vi "Find Intersections of Hyperbolas.vi"(5 "Array":T1(array[cluster]), 9 "Domain":cluster{"Start":dbl, "Stop":dbl, "Step":dbl}={"Start"=-10.0, "Stop"=10.0, "Step"=0.1}) -> ()   [LabVIEW 2013]
uses:
  <vilib>/Analysis/baseanly.llb/A x Vector.vi
  <vilib>/gmath/NI_Gmath.lvlib
  <vilib>/Analysis/NI_AALBase.lvlib
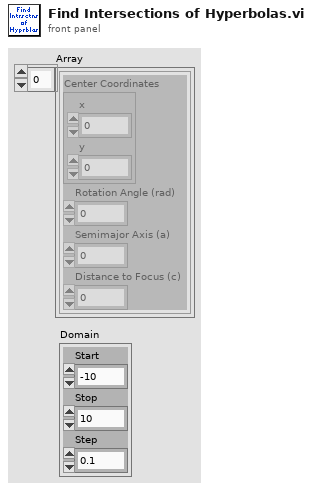
[diagram p1: front panel]
types:
  T1 = cluster{"Center Coordinates":cluster{"x":dbl, "y":dbl}, "Rotation Angle (rad)":dbl, "Semimajor Axis (a)":dbl, "Distance to Focus (c)":dbl}[]
  T2 = cluster{"A x Vector[0]":dbl, "A x Vector[1]":dbl}
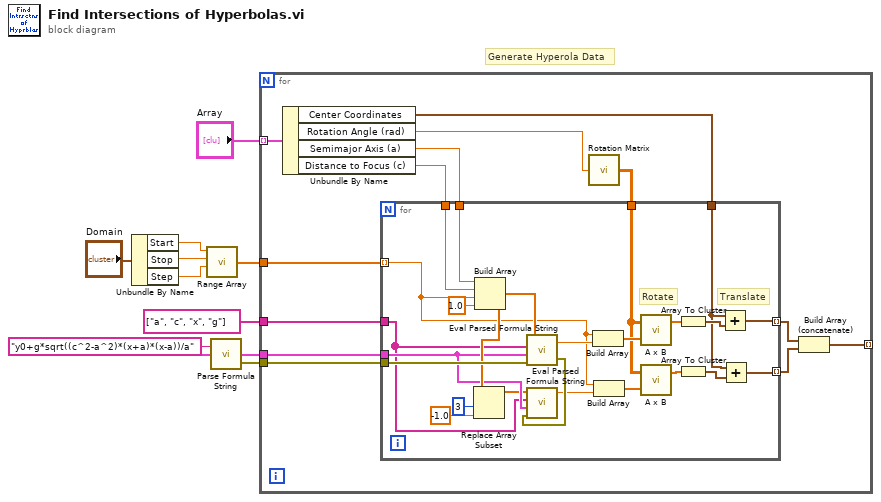
[diagram p0: block diagram]
diagram:
  # "Generate Hyperola Data"
  n1 = Unbundle By Name("Domain") -> ("Start"=w4:dbl, "Stop"=w3:dbl, "Step"=w2:dbl)
  n2 = call "Range Array.vi"("Step"=w2, "Stop"=w3, "Start"=w4) -> ("Range"=w7:dbl[])  [unwired: 3 in]
  n3 = call <vilib>:"Parse Formula String.vi"("formula"="y0+g*sqrt((c^2-a^2)*(x+a)*(x-a))/a") -> ("error out"=w10:errorcluster, "Parsed Formula"=w8:cluster{"Table":i32[][], "Y Values":dbl[]})  [unwired: 1 in]
  n4 = for {
    tunnel: w10 -> [w23]
    tunnel: w8 -> [w22]
    tunnel: w7 -> [w21]
    tunnel: string[] ["a", "c", "x", "g"] ("Variables") -> [w20]
    tunnel: [w17] -> _ mode=indexing
    tunnel: "Array" -> [w15] mode=indexing
    n5 = Unbundle By Name(w15) -> ("Center Coordinates"=w11:cluster{"x":dbl, "y":dbl}, "Rotation Angle (rad)"=w12:dbl, "Semimajor Axis (a)"=w13:dbl, "Distance to Focus (c)"=w14:dbl)
    n6 = call "Rotation Matrix.vi"("Rotation Angle (rad)"=w12) -> ("Rotation Matrix"=w16:dbl[][])  [unwired: 4 in]
    n7 = for {
      tunnel: w23 -> [w47]
      tunnel: w22 -> [w39]
      tunnel: w21 -> [w31] mode=indexing
      tunnel: w20 -> [w38]
      tunnel: w13 -> [w46]
      tunnel: w14 -> [w45]
      tunnel: w16 -> [w32]
      tunnel: [w25] -> w19 mode=indexing
      tunnel: [w26] -> w18 mode=indexing
      tunnel: w11 -> [w24]
      # "Translate"
      # "Rotate"
      n8 = Build Array(w46, w45, w31, 1.0 ("element")) -> (w43:dbl[])
      n9 = Replace Array Subset(array=w43, new element=-1.0 ("new element/subarray"), index=3) -> (w37:dbl[])
      n10 = call <vilib>:"Eval Parsed Formula String.vi"("error in (no error)"=w47, "Parsed Formula"=w39, "Variables"=w38, "X Values"=w43) -> ("error out"=w40:errorcluster, "y value"=w36:dbl)
      n11 = call <vilib>:"Eval Parsed Formula String.vi"("error in (no error)"=w40, "Parsed Formula"=w39, "Variables"=w38, "X Values"=w37) -> ("y value"=w35:dbl)  [unwired: 1 out]
      n12 = Build Array(w31, w36) -> (w34:dbl[])
      n13 = Build Array(w31, w35) -> (w33:dbl[])
      n14 = call-poly <vilib>:"A x B.vi"("Vector"=w34, "A"=w32) -> ("A x Vector"=w30:dbl[])  [unwired: 1 out]
      n15 = call-poly <vilib>:"A x B.vi"("Vector"=w33, "A"=w32) -> ("A x Vector"=w29:dbl[])  [unwired: 1 out]
      n16 = Array To Cluster(array=w30) -> (cluster=w28:T2)
      n17 = Array To Cluster(array=w29) -> (cluster=w27:T2)
      n18 = Add(x=w24, y=w28) -> (x+y=w25:cluster{dbl, dbl})
      n19 = Add(x=w24, y=w27) -> (x+y=w26:cluster{dbl, dbl})
    }
    n20 = Build Array (concatenate)(w19, w18) -> (w17:cluster{dbl, dbl}[])
  }
